vi "Read Configuration.vi"(8 "error in (no error)":errorcluster, 11 "TCP_Streamer_Subscriber in":refnum<class "TCP_Streamer_Subscriber.lvclass">) -> (0 "error out":errorcluster, 2 "Configuration":T1, 3 "TCP_Streamer_Subscriber out":refnum<class "TCP_Streamer_Subscriber.lvclass">)   [LabVIEW 2021, in "TCP_Streamer_Subscriber.lvclass"]
uses:
  TCP_Streamer_Subscriber.lvclass
  TCP_Streamer_Subscriber.lvclass/TCP_Streamer_Subscriber.ctl
  Typedef/Configuration.ctl
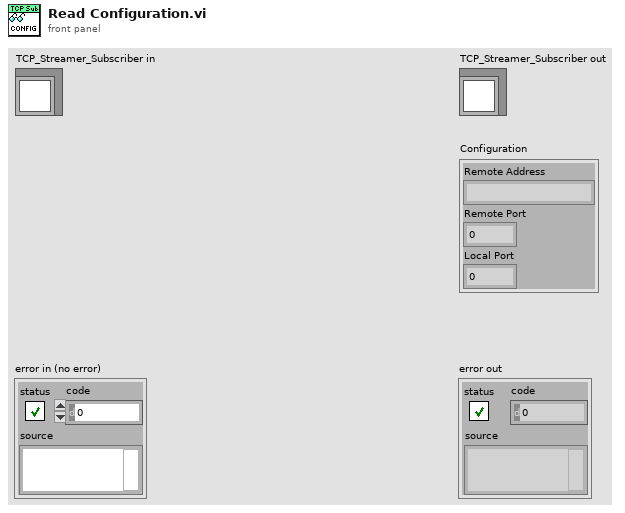
[diagram p1: front panel]
types:
  T1 = typedef "TCP_Streamer_Subscriber.lvclass/Configuration.ctl" = cluster{"Remote Address":string, "Remote Port":u16, "Local Port":u16}
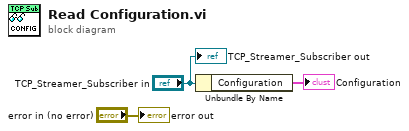
[diagram p0: block diagram]
diagram:
  n1 = Unbundle By Name("TCP_Streamer_Subscriber in") -> ("Configuration"=→"Configuration":T1)
  "error out" <- "error in (no error)"
  "TCP_Streamer_Subscriber out" <- "TCP_Streamer_Subscriber in"
